vi "Timing Report.vi"   [LabVIEW 2014]
uses:
  <vilib>/Utility/error.llb/DialogType.ctl
  <vilib>/gmath/statdist.llb/st_Percentiles (scalar).vi
  <vilib>/gmath/NI_Gmath.lvlib
  <vilib>/Wiresmith Technology/LabVIEW CLI/CLI Class/CLI.lvclass
types:
  T1 = cluster{"build_number":i32, "build_times":dbl[], "test_name":string}
  T2 = typedef "DialogType.ctl" = u16
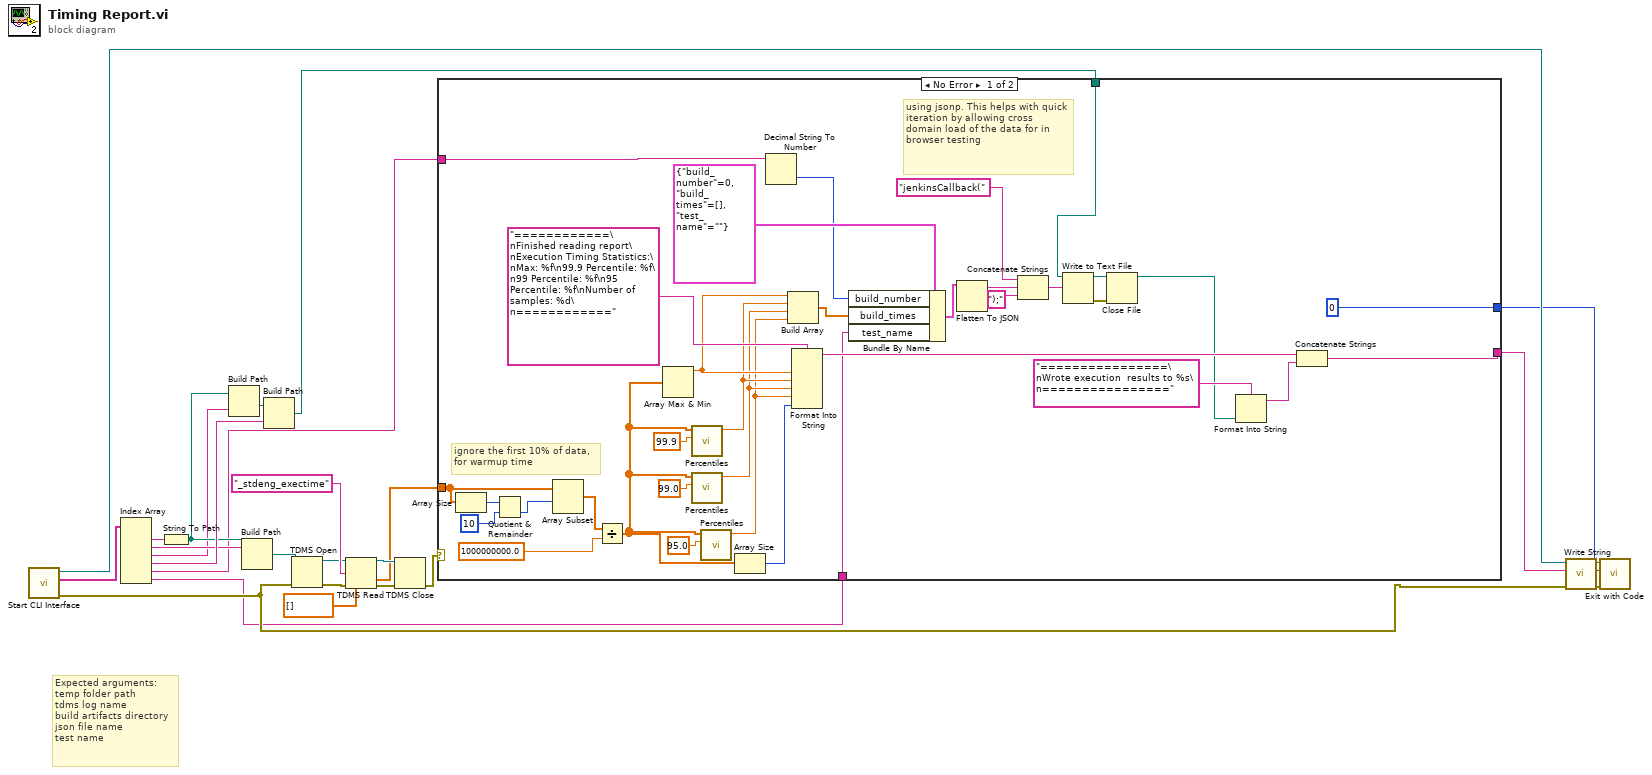
[diagram p0: block diagram]
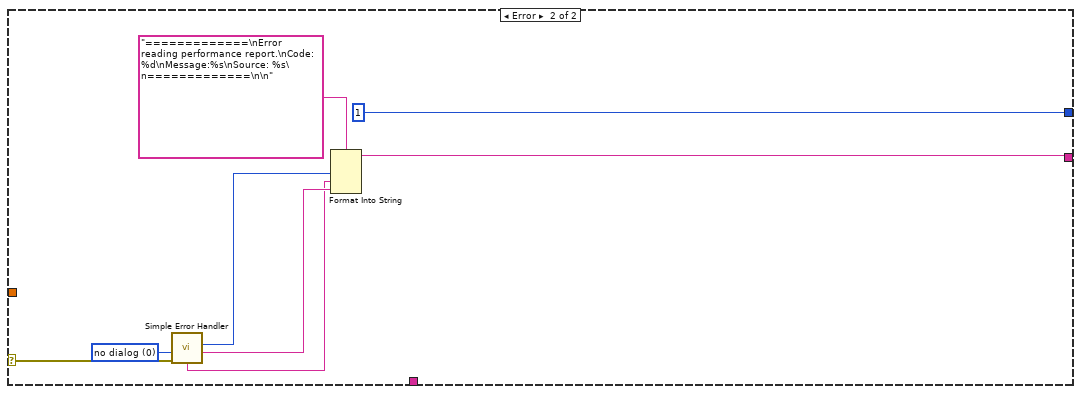
[diagram p2: hidden frame]
diagram:
  # "Expected arguments:\ntemp folder path\ntdms log name\nbuild artifacts directory\njson file name\ntest name"
  n1 = call <vilib>:"Start CLI Interface.vi"() -> ("error out"=w10:errorcluster, "Custom Parameters"=w18:string[], "CLI out"=w13:refnum<class "CLI.lvclass">)  [unwired: 9 in]
  n2 = Index Array(array=w18) -> (element #1=w17:string, element #2=w4:string, element #3=w3:string, element #4=w8:string, element #5=w2:string, element #6=w1:string)  [unwired: 6 in]
  n3 = String To Path(string=w17) -> (path=w5:path)
  n4 = Build Path(base path=w5, name or relative path=w3) -> (appended path=w6:path)
  n5 = Build Path(base path=w5, name or relative path=w4) -> (appended path=w9:path)
  n6 = Build Path(base path=w6, name or relative path=w8) -> (appended path=w7:path)
  n7 = TDMS Open(8:w10, 11:w9) -> (0:w20:errorcluster, 3:w19:refnum<k34>)  [unwired: 5 in]
  n8 = TDMS Read(0:w19, 7:"_stdeng_exectime" ("channel name(s) in"), 11:w20, 12:dbl[] []) -> (4:w25:refnum<k34>, 10:w23:dbl[], 15:w24:errorcluster)  [unwired: 4 in, 3 out]
  n9 = TDMS Close(8:w24, 11:w25) -> (0:w11:errorcluster)  [unwired: 1 out]
  n10 = case shown="No Error" w11 {
    selector: w11 -> [_ w65]
    tunnel: w23 -> [w27 _]
    tunnel: [w49 w61] -> w14
    tunnel: [0 ("Exit Code (0)") 1 ("Exit Code (0)")] -> w12
    tunnel: w7 -> [w46 _]
    tunnel: w2 -> [w38 _]
    tunnel: w1 -> [w31 _]
    frame No Error {
      # "ignore the first 10% of data,\nfor warmup time"
      # "using jsonp. This helps with quick iteration by allowing cross domain load of the data for in browser testing"
      n11 = Array Size(array=w27) -> (size(s)=w30:i32)
      n12 = Quotient & Remainder(x=w30, y=10) -> (floor(x/y)=w28:i32)  [unwired: 1 out]
      n13 = Array Subset(array=w27, index=w28) -> (w26:dbl[])  [unwired: 1 in]
      n14 = Divide(x=w26, y=1000000000.0) -> (x/y=w33:dbl[])
      n15 = Array Max & Min(array=w33) -> (max value=w54:dbl)  [unwired: 3 out]
      n16 = call-poly <vilib>:"Percentiles.vi"("p"=99.9, "x array"=w33) -> ("percentile"=w53:dbl)  [unwired: 8 in, 1 out]
      n17 = call-poly <vilib>:"Percentiles.vi"("p"=99.0, "x array"=w33) -> ("percentile"=w52:dbl)  [unwired: 8 in, 1 out]
      n18 = call-poly <vilib>:"Percentiles.vi"("p"=95.0, "x array"=w33) -> ("percentile"=w51:dbl)  [unwired: 8 in, 1 out]
      n19 = Array Size(array=w33) -> (size(s)=w32:i32)
      n20 = Decimal String To Number(string=w38) -> (number=w36:i32)  [unwired: 2 in, 1 out]
      n21 = Build Array(w54, w53, w52, w51) -> (w35:dbl[])
      n22 = Format Into String(format string="============\nFinished reading report\nExecution Timing Statistics:\nMax: %f\n99.9 Percentile: %f\n99 Percentile: %f\n95 Percentile: %f\nNumber of samples: %d\n============", w54, w53, w52, w51, w32) -> (resulting string=w48:string)  [unwired: 2 in, 1 out]
      n23 = Bundle By Name(cluster=T1 {"build_number"=0, "build_times"=[], "test_name"=""}, "build_number"=w36, "build_times"=w35, "test_name"=w31) -> (w34:T1)
      n24 = Flatten To JSON(anything=w34) -> (JSON string=w41:string)  [unwired: 2 in, 1 out]
      n25 = Concatenate Strings("jenkinsCallback(" ("string"), w41, ");" ("string")) -> (w42:string)
      n26 = Write to Text File(file (use dialog)=w46, text=w42) -> (refnum out=w44:refnum<file>, error out=w45:errorcluster)  [unwired: 2 in, 1 out]
      n27 = Close File(refnum=w44, error in=w45) -> (path=w43:path)  [unwired: 1 out]
      n28 = Format Into String(format string="================\nWrote execution  results to %s\n================", w43) -> (resulting string=w47:string)  [unwired: 2 in, 1 out]
      n29 = Concatenate Strings(w48, w47) -> (w49:string)
    }
    frame Error {
      w66 = T2 0 items=["no dialog", "OK message", "continue or stop message", "OK message + warnings", "continue/stop + warnings"] ("type of dialog (OK msg:1)")
      n30 = call <vilib>:"Simple Error Handler.vi"("type of dialog (OK msg:1)"=w66, "error in (no error)"=w65) -> ("code out"=w64:i32, "source out"=w63:string, "message"=w62:string)  [unwired: 3 in, 2 out]
      n31 = Format Into String(format string="=============\nError reading performance report.\nCode: %d\nMessage:%s\nSource: %s\n=============\n\n", w64, w62, w63) -> (resulting string=w61:string)  [unwired: 2 in, 1 out]
    }
  }
  n32 = call <vilib>:"Write String.vi"("error in (no error)"=w10, "Text to Write"=w14, "CLI in"=w13) -> ("error out"=w16:errorcluster, "CLI out"=w15:refnum<class "CLI.lvclass">)  [unwired: 7 in]
  n33 = call <vilib>:"Exit with Code.vi"("error in (no error)"=w16, "Exit Code (0)"=w12, "CLI in"=w15) -> ()  [unwired: 8 in, 1 out]
